vi "BuckConverterGraphData.vi"(7 "LabVIEW Web Service Request":refnum<class "Web Request.lvclass">) -> ()   [LabVIEW 2015]
uses:
  <vilib>/wsapi/Web Request.lvclass
  <vilib>/imath/engines/lvmath2/RunTimeEngine/Managers/WorkSpace/UID Generator.vi
  <vilib>/imath/engines/lvmath/Plug In/Control Design/BuiltInFunctions/tf/NIMS_CD_tf(STR,Ts).vi
  <vilib>/imathl/engines/lvmath/Functions/Error Handling/Create Error.vi
  <vilib>/imath/engines/lvmath/Plug In/Control Design/BuiltInFunctions/multmx/NIMS_CD_multmx(TF,K).vi
  <vilib>/imath/engines/lvmath/Plug In/Control Design/BuiltInFunctions/plus/NIMS_CD_plus(K,TF).vi
  <vilib>/imath/engines/lvmath/Functions/Error Handling/MergeErrorsWrapper.vi
  <vilib>/imath/engines/lvmath/Plug In/Control Design/BuiltInFunctions/powermx/NIMS_CD_powermx(TF,N).vi
  <vilib>/imath/engines/lvmath/Plug In/Control Design/BuiltInFunctions/plus/NIMS_CD_plus(TF,TF).vi
  <vilib>/imath/engines/lvmath/Plug In/Control Design/BuiltInFunctions/rightdivmx/NIMS_CD_rightdivmx(TF,TF).vi
  <vilib>/imath/engines/lvmath2/RunTimeEngine/RunTimeType/NIMS_RunTimeType_From StrictType (excl LVString).vi
  <instcachedir>/0/NIMS_RunTimeType_From StrictType (excl LVString)_EB1C38A9BC5048DA9ABDA8F781E54D21.lvgen/NIMS_RunTimeType_From StrictType (excl LVString)_EB1C38A9BC5048DA9ABDA8F781E54D21_031.vi
  <vilib>/imath/engines/lvmath2/RunTimeEngine/LocalVariableDefStatement/MC_LocalVariableDefStatement_Display.vi
  <vilib>/imath/engines/lvmath/Plug In/Control Design/BuiltInFunctions/multmx/NIMS_CD_multmx(K,TF).vi
  <vilib>/imath/engines/lvmath/Plug In/Control Design/BuiltInFunctions/rightdivmx/NIMS_CD_rightdivmx(TF,K).vi
  <vilib>/imath/engines/lvmath/Plug In/Control Design/BuiltInFunctions/step/NIMS_CD_[Y,T]=step(TF,[Tinfo]).vi
  <vilib>/imath/engines/lvmath2/RunTimeEngine/Managers/SymbolTable/Clear UID.vi
  <vilib>/imath/engines/lvmath2/RunTimeEngine/NodeEndStatement/NIMS_NodeEndStatement_Output.vi
  <instcachedir>/0/NIMS_NodeEndStatement_Output_53EC0D466D134D7ABD903AC30B43404B.lvgen/NIMS_NodeEndStatement_Output_53EC0D466D134D7ABD903AC30B43404B_002.vi
  <vilib>/imath/engines/lvmath2/RunTimeEngine/ErrorHandling/NIMS_Finalize Error.vi
  <vilib>/Analysis/Matrix/Numeric/Conversions/Matrix To Array.vi
  <vilib>/Analysis/Matrix/Numeric/Conversions/Matrix To Array - RM.vi
  <vilib>/Analysis/Matrix/NI_Matrix.lvlib
  <vilib>/imath/engines/lvmath2/RunTimeEngine/Managers/SymbolTable/NIMS_WorkSpace.lvlib
panel:
  out "Waveform Graph 2":dbl[](graph)
  out "[0]":i32
  out "error out":errorcluster
  out "JSON string":string
  in  "error in (no error)":errorcluster
  # "Use the Web Service Request input terminal to call the VIs on the Web Services palette. Do not remove it from the connector pane unless you don't need access to the palette."
  # "Each additional control wired to the connector pane will be available as an input in the URL. To include an indicator in terminal-mode output (the default setting), it must also be wired to the connector pane."
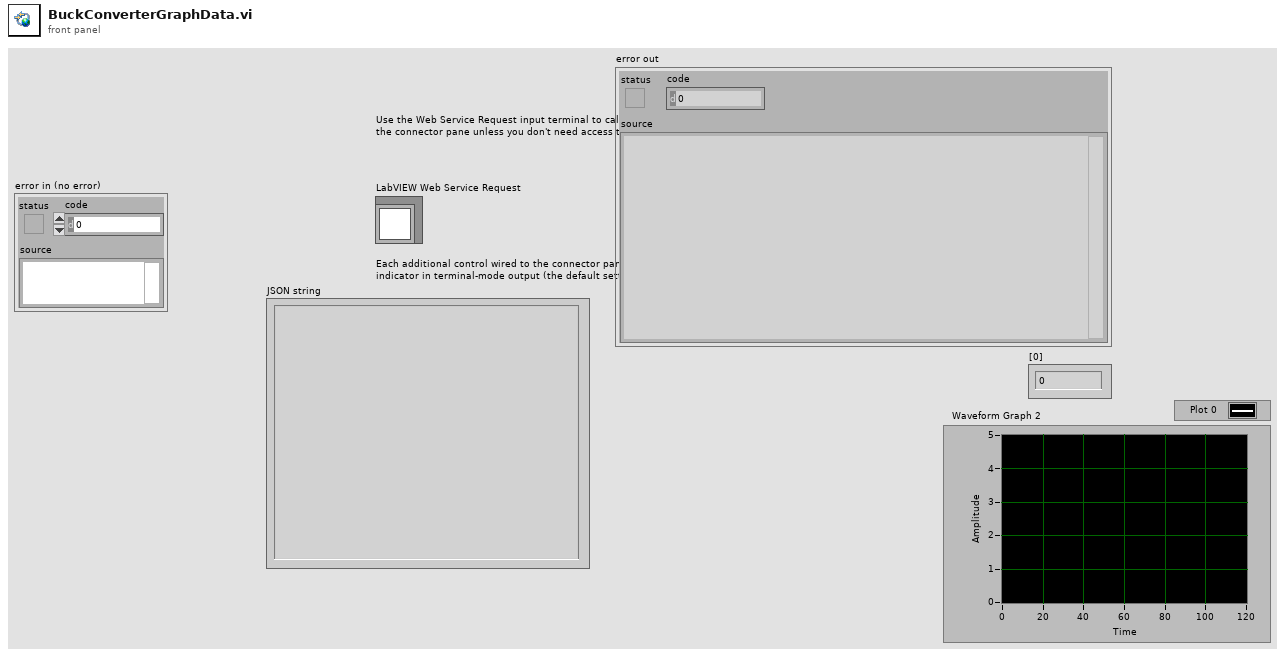
[diagram p1: front panel]
types:
  T1 = cluster{"[0]":i32, "[1]":i32, "[2]":i32, "[3]":i32, "[4]":i32}
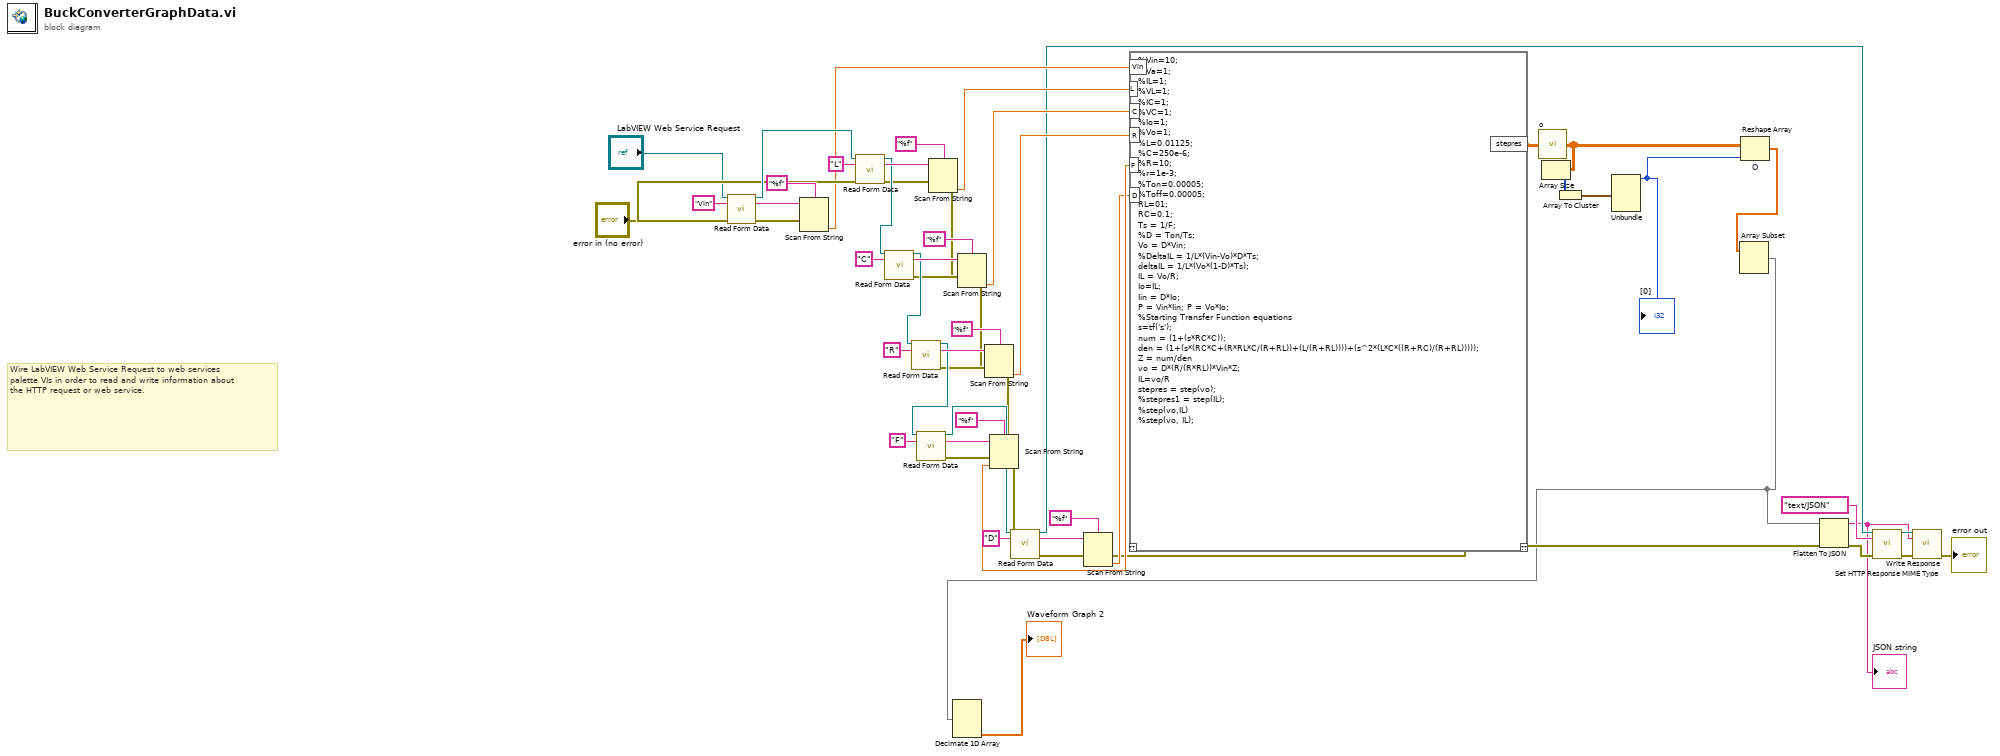
[diagram p0: block diagram]
diagram:
  # "Wire LabVIEW Web Service Request to web services palette VIs in order to read and write information about the HTTP request or web service."
  n1 = call <vilib>:"Read Form Data.vi"("LabVIEW Web Service Request"="LabVIEW Web Service Request", "key"="Vin", "error in (no error)"="error in (no error)") -> ("LabVIEW Web Service Request out"=w53:refnum<class "Web Request.lvclass">, "value"=w56:string, "error out"=w24:errorcluster)  [unwired: 9 in, 1 out]
  n2 = Scan From String(format string="%f", input string=w56, error in=w24) -> (error out=w25:errorcluster, output 1=w22:dbl)  [unwired: 2 in, 2 out]
  n3 = call <vilib>:"Read Form Data.vi"("LabVIEW Web Service Request"=w53, "key"="L", "error in (no error)"=w25) -> ("LabVIEW Web Service Request out"=w48:refnum<class "Web Request.lvclass">, "value"=w54:string, "error out"=w26:errorcluster)  [unwired: 9 in, 1 out]
  n4 = Scan From String(format string="%f", input string=w54, error in=w26) -> (error out=w27:errorcluster, output 1=w21:dbl)  [unwired: 2 in, 2 out]
  n5 = call <vilib>:"Read Form Data.vi"("LabVIEW Web Service Request"=w48, "key"="C", "error in (no error)"=w27) -> ("LabVIEW Web Service Request out"=w44:refnum<class "Web Request.lvclass">, "value"=w50:string, "error out"=w28:errorcluster)  [unwired: 9 in, 1 out]
  n6 = Scan From String(format string="%f", input string=w50, error in=w28) -> (error out=w29:errorcluster, output 1=w20:dbl)  [unwired: 2 in, 2 out]
  n7 = call <vilib>:"Read Form Data.vi"("LabVIEW Web Service Request"=w44, "key"="R", "error in (no error)"=w29) -> ("LabVIEW Web Service Request out"=w40:refnum<class "Web Request.lvclass">, "value"=w46:string, "error out"=w30:errorcluster)  [unwired: 9 in, 1 out]
  n8 = Scan From String(format string="%f", input string=w46, error in=w30) -> (error out=w31:errorcluster, output 1=w14:dbl)  [unwired: 2 in, 2 out]
  n9 = call <vilib>:"Read Form Data.vi"("LabVIEW Web Service Request"=w40, "key"="F", "error in (no error)"=w31) -> ("LabVIEW Web Service Request out"=w36:refnum<class "Web Request.lvclass">, "value"=w42:string, "error out"=w32:errorcluster)  [unwired: 9 in, 1 out]
  n10 = Scan From String(format string="%f", input string=w42, error in=w32) -> (error out=w33:errorcluster, output 1=w19:dbl)  [unwired: 2 in, 2 out]
  n11 = call <vilib>:"Read Form Data.vi"("LabVIEW Web Service Request"=w36, "key"="D", "error in (no error)"=w33) -> ("LabVIEW Web Service Request out"=w12:refnum<class "Web Request.lvclass">, "value"=w38:string, "error out"=w34:errorcluster)  [unwired: 9 in, 1 out]
  n12 = Scan From String(format string="%f", input string=w38, error in=w34) -> (error out=w11:errorcluster, output 1=w18:dbl)  [unwired: 2 in, 2 out]
  n13 = mathscript code="%Vin=10;\n%Va=1;\n%IL=1;\n%VL=1;\n%IC=1;\n%VC=1;\n%Io=1;\n%Vo=1;\n%L=0.01125;\n%C=250e-6;\n%R=10;\n%r=1e-3;\n%Ton=0.00005;\n%Toff=0.00005;\nRL=01;\nRC=0.1;\nTs = 1/F;\n%D = Ton/Ts;\nVo = D*Vin;\n%DeltaIL = 1/L*(Vin-Vo)*D*Ts;\ndeltaIL = 1/L*(Vo*(1-D)*Ts);\nIL = Vo/R;\nIo=IL;\nIin = D*Io;\nP = Vin*Iin; P = Vo*Io;\n%Starting Transfer Function equations\ns=tf('s');\nnum = (1+(s*RC*C));\nden = (1+(s*(RC*C+(R*RL*C/(R+RL))+(L/(R+RL))))+(s^2*(L*C*((R+RC)/(R+RL)))));\nZ = num/den\nvo = D*(R/(R*RL))*Vin*Z;\nIL=vo/R\nstepres = step(vo);\n%stepres1 = step(IL);\n%step(vo,IL)\n%step(vo, IL);"("Vin"=w22, "L"=w21, "C"=w20, "R"=w14, "F"=w19, "D"=w18) -> ("stepres"=w7:dbl[][])  [unwired: 1 in, 1 out]
  n14 = call-poly "o"("Real Matrix"=w7) -> ("Real 2D Array"=w5:dbl[][])
  n15 = Array Size(array=w5) -> (size(s)=w9:i32[])
  n16 = Array To Cluster(array=w9) -> (cluster=w8:T1)
  n17 = Unbundle(w8) -> ("[0]"=w4:i32)  [unwired: 4 out]
  "[0]" <- w4
  n18 = Reshape Array "O"(w5, w4) -> (w3:dbl[])
  n19 = Array Subset(array=w3) -> (w1:dbl[])  [unwired: 2 in]
  n20 = Decimate 1D Array(w1) -> (→"Waveform Graph 2":dbl[])  [unwired: 4 out]
  n21 = Flatten To JSON(anything=w1, error in (no error)=w11) -> (JSON string=w6:string, 11:w13:errorcluster)  [unwired: 1 in]
  "JSON string" <- w6
  n22 = call <vilib>:"Set HTTP Response MIME Type.vi"("LabVIEW Web Service Request"=w12, "MIME type (text/html)"="text/JSON", "error in (no error)"=w13) -> ("LabVIEW Web Service Request out"=w17:refnum<class "Web Request.lvclass">, "error out"=w16:errorcluster)  [unwired: 11 in]
  n23 = call <vilib>:"Write Response.vi"("LabVIEW Web Service Request"=w17, "response string"=w6, "error in (no error)"=w16) -> ("error out"=→"error out":errorcluster)  [unwired: 11 in, 1 out]
